vi "ROI entry-Initialisation26_01_18.vi"(9 "Pane refs array":refnum<vi>[](array[refnum]), 11 "User Events Cluster":T1) -> (3 "Open file dialogue window":bool)   [LabVIEW 2020]
uses:
  Typedefs/ROI management FG states.ctl
  Typedefs/Save-Load enum.ctl
  Global Variables/General Globals.vi
  Typedefs/Offsets cluster.ctl
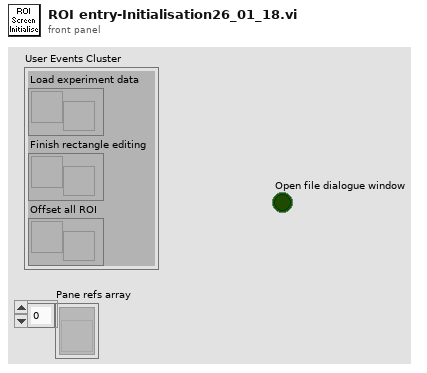
[diagram p1: front panel]
types:
  T1 = cluster{"Load experiment data":refnum<user-event>, "Finish rectangle editing":refnum<user-event>, "Offset all ROI":refnum<user-event>}
  T2 = typedef "ROI management FG states.ctl" = enum16{"Read", "Write", "Write-from dataset", "Clear Last", "Clear All", "Delete ROI", "Update ROIs time", "Reload last ROI set", "Modify ROI Parameters", "Offset all ROI", "Offset visible ROI", "Modify Dwell Time", "Modify Laser Power"}
  T3 = typedef "Save-Load enum.ctl" = enum16{"Save to file", "Load from file", "Compare from file", "Save Backup"}
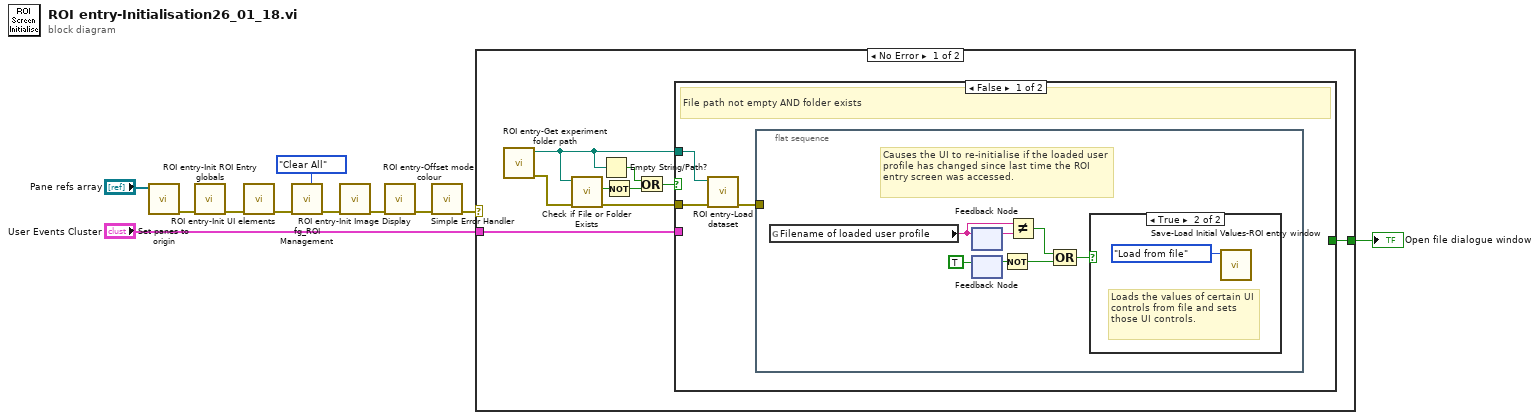
[diagram p0: block diagram]
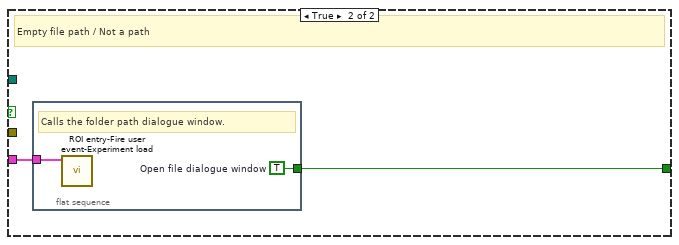
[diagram p3: hidden frame]
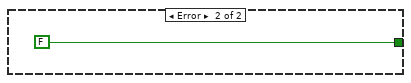
[diagram p4: hidden frame]
diagram:
  n1 = call "Set panes to origin.vi"("Pane refs array"="Pane refs array") -> ("error out"=w6:errorcluster)  [unwired: 10 in]
  n2 = call "ROI entry-Init ROI Entry globals.vi"("error in (no error)"=w6) -> ("error out"=w5:errorcluster)  [unwired: 10 in]
  n3 = call "ROI entry-Init UI elements.vi"("error in (no error)"=w5) -> ("error out"=w7:errorcluster)  [unwired: 10 in]
  n4 = call "fg_ROI Management.vi"("Function"=ROI_management_FG_states."Clear All", "error in (no error)"=w7) -> ("error out"=w8:errorcluster)  [unwired: 5 in, 4 out]
  n5 = call "ROI entry-Init Image Display.vi"("error in (no error)"=w8) -> ("error out"=w2:errorcluster)  [unwired: 10 in]
  n6 = call "ROI entry-Offset mode colour.vi"("error in (no error)"=w2) -> ("error out"=w1:errorcluster)  [unwired: 10 in]
  n7 = call <vilib>:"Simple Error Handler.vi"("error in (no error)"=w1) -> ("error out"=w4:errorcluster)  [unwired: 4 in, 4 out]
  n8 = case shown="No Error" w4 {
    tunnel: "User Events Cluster" -> [w19 _]
    tunnel: [w18 FALSE ("Open file dialogue window")] -> w10
    frame No Error {
      n9 = call "ROI entry-Get experiment folder path.vi"() -> ("error out"=w12:errorcluster, "Experiment folder path"=w13:path)  [unwired: 10 in]
      n10 = call <vilib>:"Check if File or Folder Exists.vi"("error in (no error)"=w12, "path"=w13) -> ("error out"=w20:errorcluster, "file or folder exists?"=w14:bool)  [unwired: 7 in, 1 out]
      n11 = Empty String/Path?(string/path=w13) -> (empty?=w16:bool)
      n12 = Not(x=w14) -> (.not. x?=w15:bool)
      n13 = Or(x=w16, y=w15) -> (x .or. y?=w17:bool)
      n14 = case shown="False" w17 {
        tunnel: w13 -> [w23 _]
        tunnel: w19 -> [_ w33]
        tunnel: [_ w32] -> w18
        tunnel: w20 -> [w22 _]
        frame False {
          # "File path not empty AND folder exists"
          n15 = call "ROI entry-Load dataset.vi"("error in (no error)"=w22, "Experiment folder path OR Z-stack folder path"=w23) -> ("error out"=w21:errorcluster)  [unwired: 9 in]
          n16 = flat-sequence {
            tunnel: w21 -> [_]
            frame #0 {
              # "Causes the UI to re-initialise if the loaded user profile has changed since last time the ROI entry screen was accessed."
              n17 = global read "General Globals.vi" "Filename of loaded user profile"() -> (w27:string)
              n18 = feedback #1() -> (w28:string)  [unwired: 1 in]
              n19 = feedback-in #1(w27) -> ()
              n20 = feedback #2() -> (w30:bool)  [unwired: 1 in]
              n21 = feedback-in #2(TRUE) -> ()
              n22 = Not(x=w30) -> (.not. x?=w26:bool)
              n23 = Not Equal?(x=w27, y=w28) -> (x != y?=w24:bool)
              n24 = Compound Arithmetic op=OR(w24, w26) -> (w25:bool)
              n25 = case shown="True" w25 {
                frame False {
                }
                frame True {
                  # "Loads the values of certain UI controls from file and sets those UI controls."
                  n26 = call "Save-Load Initial Values-ROI entry window.vi"("Function"=Save-Load_enum."Load from file") -> ()  [unwired: 10 in, 1 out]
                }
              }
            }
          }
        }
        frame True {
          # "Empty file path / Not a path"
          n27 = flat-sequence {
            tunnel: w33 -> [w34]
            tunnel: [w35] -> w32
            frame #0 {
              w35 = TRUE  # Open file dialogue window
              # "Calls the folder path dialogue window."
              n28 = call "ROI entry-Fire user event-Experiment load.vi"("User Events Cluster"=w34) -> ()  [unwired: 10 in, 1 out]
            }
          }
        }
      }
    }
    frame Error {
    }
  }
  "Open file dialogue window" <- w10
